vi "read_s7_1200 (SubVI).vi"(8 "error in (no error)":errorcluster, 11 "Refnum in":T1) -> (0 "error out":errorcluster, 1 "VALUES READ":map{string, i32}(c390), 2 "Coils read":map{string, bool}(c390), 3 "Refnum out":T1)   [LabVIEW 2024]
uses:
  <vilib>/OPCUA/controls/OPC UA Client Refnum.ctl
  <vilib>/OPCUA/controls/NodeIds.ctl
  <vilib>/OPCUA/controls/NodeId.ctl
  <vilib>/OPCUA/client/Multiple Read Bool.vi
  <vilib>/OPCUA/client/Multiple Read UInt16.vi
  <vilib>/OPCUA/NI OPC UA Client.lvlib
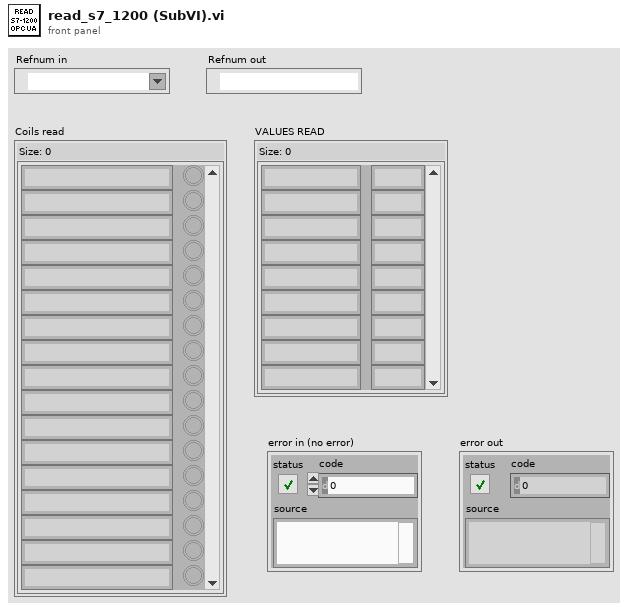
[diagram p1: front panel]
types:
  T1 = typedef "OPC UA Client Refnum.ctl" = refnum<k21>
  T2 = typedef "NodeIds.ctl" = T3[]
  T3 = typedef "NodeId.ctl" = string
  T4 = typedef "OPC UA StatusCode.ctl" = u32
  T5 = cluster{"node ID":T3, "value ":bool, "timestamp":timestamp, "status":T4}[]
  T6 = cluster{"node ID":T3, "value ":u16, "timestamp":timestamp, "status":T4}[]
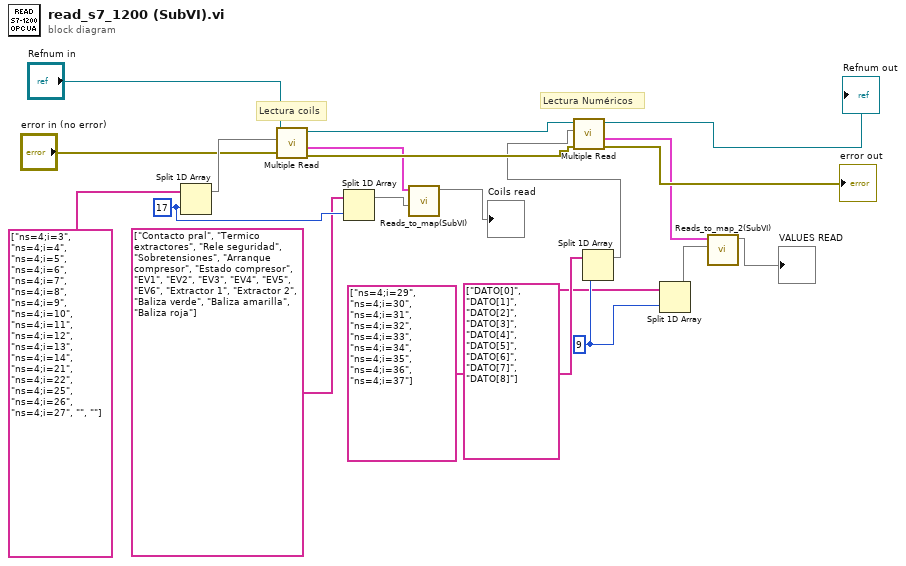
[diagram p0: block diagram]
diagram:
  w16 = 9 ("index")
  w8 = 17 ("index")
  # "Lectura Numéricos"
  # "Lectura coils"
  n1 = Split 1D Array(array=T2 ["ns=4;i=3", "ns=4;i=4", "ns=4;i=5", "ns=4;i=6", "ns=4;i=7", "ns=4;i=8", "ns=4;i=9", "ns=4;i=10", "ns=4;i=11", "ns=4;i=12", "ns=4;i=13", "ns=4;i=14", "ns=4;i=21", "ns=4;i=22", "ns=4;i=25", "ns=4;i=26", "ns=4;i=27", "", ""] ("node IDs"), index=w8) -> (first subarray=w6:T2)  [unwired: 1 out]
  n2 = call-poly <vilib>:"Multiple Read.vi"("error in (no error)"="error in (no error)", "node IDs"=w6, "OPC UA client refnum in"="Refnum in") -> ("error out"=w19:errorcluster, "results"=w3:T5, "OPC UA client refnum out"=w10:T1)  [unwired: 5 in, 1 out]
  n3 = Split 1D Array(array=string[] ["Contacto pral", "Termico extractores", "Rele seguridad", "Sobretensiones", "Arranque compresor", "Estado compresor", "EV1", "EV2", "EV3", "EV4", "EV5", "EV6", "Extractor 1", "Extractor 2", "Baliza verde", "Baliza amarilla", "Baliza roja"], index=w8) -> (first subarray=w9:string[])  [unwired: 1 out]
  n4 = call "Reads_to_map(SubVI).vi"("Key Array"=w9, "Read Input Cluster"=w3) -> ("Output map"=→"Coils read":map{string, bool})  [unwired: 9 in]
  n5 = Split 1D Array(array=T2 ["ns=4;i=29", "ns=4;i=30", "ns=4;i=31", "ns=4;i=32", "ns=4;i=33", "ns=4;i=34", "ns=4;i=35", "ns=4;i=36", "ns=4;i=37"] ("node IDs"), index=w16) -> (first subarray=w17:T2)  [unwired: 1 out]
  n6 = call-poly <vilib>:"Multiple Read.vi"("error in (no error)"=w19, "node IDs"=w17, "OPC UA client refnum in"=w10) -> ("error out"=→"error out":errorcluster, "results"=w12:T6, "OPC UA client refnum out"=→"Refnum out":T1)  [unwired: 5 in, 1 out]
  n7 = Split 1D Array(array=string[] ["DATO[0]", "DATO[1]", "DATO[2]", "DATO[3]", "DATO[4]", "DATO[5]", "DATO[6]", "DATO[7]", "DATO[8]"] ("Key Array"), index=w16) -> (first subarray=w18:string[])  [unwired: 1 out]
  n8 = call "Reads_to_map_2(SubVI).vi"("Key Array"=w18, "results"=w12) -> ("Map"=→"VALUES READ":map{string, i32})  [unwired: 9 in]
